vi "Error Converter (ErrCode or Status).vi"(8 "error in (no error)":errorcluster, 11 "error code":i32) -> (0 "error out":errorcluster)   [LabVIEW 2013]
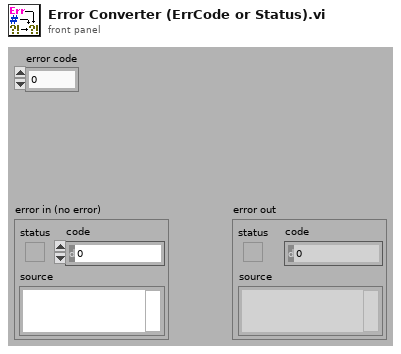
[diagram p1: front panel]
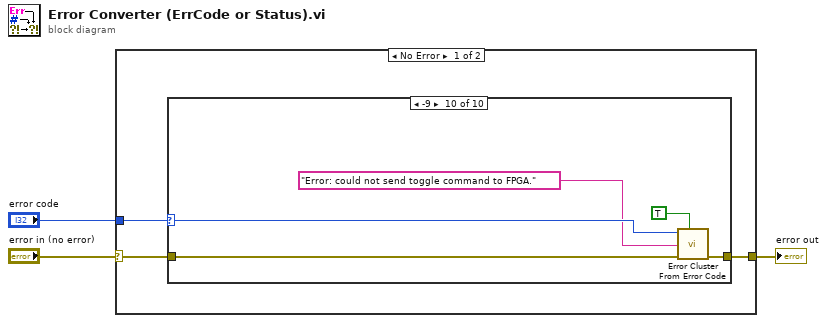
[diagram p0: block diagram]
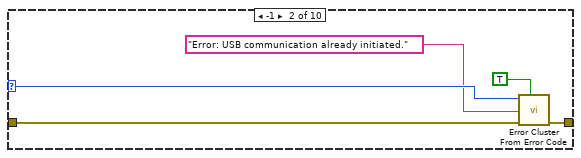
[diagram p3: hidden frame]
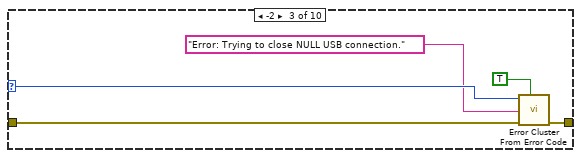
[diagram p4: hidden frame]
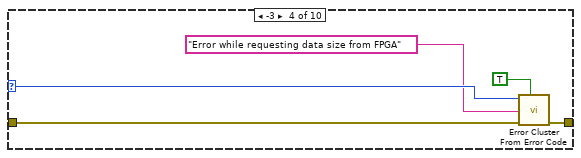
[diagram p5: hidden frame]
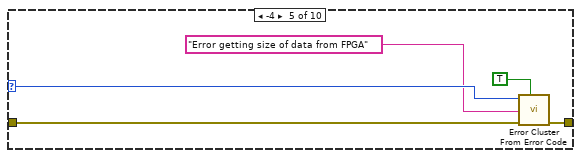
[diagram p6: hidden frame]
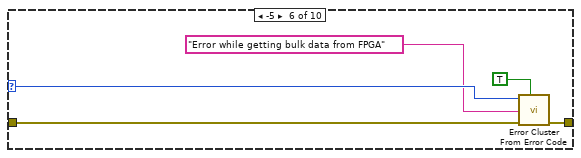
[diagram p7: hidden frame]
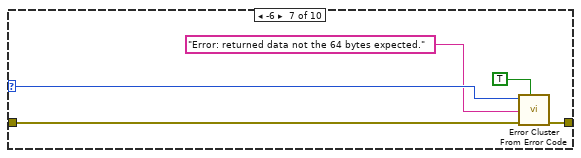
[diagram p8: hidden frame]
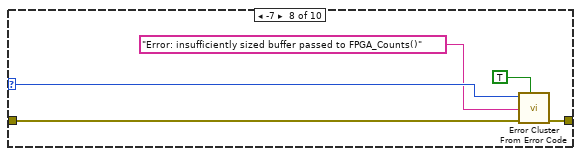
[diagram p9: hidden frame]
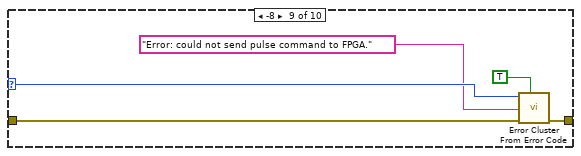
[diagram p10: hidden frame]
diagram:
  n1 = case shown="No Error" "error in (no error)" {
    selector: "error in (no error)" -> [w6 w53]
    tunnel: [w5 w53] -> w2
    tunnel: "error code" -> [w4 _]
    frame No Error {
      n2 = case shown="-9" w4 {
        selector: w4 -> [_ w9 w14 w19 w24 w29 w34 w39 w44 w49]
        tunnel: w6 -> [w7 w12 w17 w22 w27 w32 w37 w42 w47 w52]
        tunnel: [w7 w11 w16 w21 w26 w31 w36 w41 w46 w51] -> w5
        frame 0, Default {
        }
        frame -1 {
          n3 = call <vilib>:"Error Cluster From Error Code.vi"("show call chain? (False)"=TRUE, "error in (no error)"=w12, "error message (\"\")"="Error: USB communication already initiated.", "error code (0)"=w9) -> ("error out"=w11:errorcluster)  [unwired: 5 in]
        }
        frame -2 {
          n4 = call <vilib>:"Error Cluster From Error Code.vi"("show call chain? (False)"=TRUE, "error in (no error)"=w17, "error message (\"\")"="Error: Trying to close NULL USB connection.", "error code (0)"=w14) -> ("error out"=w16:errorcluster)  [unwired: 5 in]
        }
        frame -3 {
          n5 = call <vilib>:"Error Cluster From Error Code.vi"("show call chain? (False)"=TRUE, "error in (no error)"=w22, "error message (\"\")"="Error while requesting data size from FPGA", "error code (0)"=w19) -> ("error out"=w21:errorcluster)  [unwired: 5 in]
        }
        frame -4 {
          n6 = call <vilib>:"Error Cluster From Error Code.vi"("show call chain? (False)"=TRUE, "error in (no error)"=w27, "error message (\"\")"="Error getting size of data from FPGA", "error code (0)"=w24) -> ("error out"=w26:errorcluster)  [unwired: 5 in]
        }
        frame -5 {
          n7 = call <vilib>:"Error Cluster From Error Code.vi"("show call chain? (False)"=TRUE, "error in (no error)"=w32, "error message (\"\")"="Error while getting bulk data from FPGA", "error code (0)"=w29) -> ("error out"=w31:errorcluster)  [unwired: 5 in]
        }
        frame -6 {
          n8 = call <vilib>:"Error Cluster From Error Code.vi"("show call chain? (False)"=TRUE, "error in (no error)"=w37, "error message (\"\")"="Error: returned data not the 64 bytes expected.", "error code (0)"=w34) -> ("error out"=w36:errorcluster)  [unwired: 5 in]
        }
        frame -7 {
          n9 = call <vilib>:"Error Cluster From Error Code.vi"("show call chain? (False)"=TRUE, "error in (no error)"=w42, "error message (\"\")"="Error: insufficiently sized buffer passed to FPGA_Counts()", "error code (0)"=w39) -> ("error out"=w41:errorcluster)  [unwired: 5 in]
        }
        frame -8 {
          n10 = call <vilib>:"Error Cluster From Error Code.vi"("show call chain? (False)"=TRUE, "error in (no error)"=w47, "error message (\"\")"="Error: could not send pulse command to FPGA.", "error code (0)"=w44) -> ("error out"=w46:errorcluster)  [unwired: 5 in]
        }
        frame -9 {
          n11 = call <vilib>:"Error Cluster From Error Code.vi"("show call chain? (False)"=TRUE, "error in (no error)"=w52, "error message (\"\")"="Error: could not send toggle command to FPGA.", "error code (0)"=w49) -> ("error out"=w51:errorcluster)  [unwired: 5 in]
        }
      }
    }
    frame Error {
    }
  }
  "error out" <- w2
